vi "Do_Offset.vi"(0 "VRN IN":refnum<visa-resource-name>[](array[refnum])=["-1", "-1"] caption="VRN IN [TCS, Table, Prams]", 1 "TCS Actif":refnum<vi>, 2 "Table_Astrom":T2={"NAXIS"=[1000000.0, 1000000.0], "CD"=[[7.753782961940616e-07, 4.45891648260791e-07], [4.45891648260791e-07, -7.753782961940616e-07]], "CDELT"=[1.0, 1.0], "CRPIX"=[669354.0, 53563.0], "CTYPE"=["RA---TAN", "DEC--TAN"], "CRVAL"=[53.2938, 45.43681200000001], "LONGPOLE"=180.0, "LATPOLE"=90.0, "PV2"=[0.0, 0.0]} {"CRVAL" format="%.6g"; "CD" format="%_7g"}, 5 "RA offset":dbl format="%.2f", 9 "DEC offset":dbl format="%.2f", 11 "Error IN":errorcluster[](array[cluster])=[{"status"=FALSE, "code"=0, "source"=""}, {"status"=FALSE, "code"=0, "source"=""}] caption="Error IN [TCS C, Table]", 13 "Field_Astrom":T2 {"CRVAL" format="%.6g"; "CD" format="%_7g"}) -> (4 "VRN OUT":refnum<visa-resource-name>[](array[refnum]) caption="VRN OUT [TCS C, Table, Prams]", 6 "Error code":u8, 8 "Undo offset":bool, 10 "Warning code":u8, 14 "Error Comment":string, 15 "Error OUT":errorcluster[](array[cluster]) caption="Error OUT [TCS C, Table]")   [LabVIEW 2011]
uses:
  Globals.vi
  Polymorphics/Distance(array).vi
panel:
  out "BooleanReferences":T1
  out "Prams Error":errorcluster
  out "Table Error":errorcluster
  out "TCS Error":errorcluster
  in  "Prams VRN":refnum<visa-resource-name>
  in  "Table VRN":refnum<visa-resource-name>
  in  "TCS VRN":refnum<visa-resource-name>
  in  "Prams ACK":refnum<vi>
  in  "Prams Actif":refnum<vi>
  in  "Table Actif":refnum<vi>
  in  "FOV":dbl format="%.2f"
  in  "EPOCH":dbl format="%.2f"
  out "RA after":dbl
  out "DEC after":dbl
  in  "USNO_data":string[][](array[string])
  out "New Source Found ?":bool
  out "cible Y":dbl
  out "cible X":dbl
  out "Accesible?":bool
  out "DEC Goffset":dbl=10.0 format="%.2f"
  out "RA Goffset":dbl=10.0 format="%.2f"
  out "DEC Moffset":dbl format="%.2f"
  out "RA Moffset":dbl format="%.2f"
  out "Guiding":bool caption="Guider was running"
  out "Moffset":bool
  out "Goffset":bool
  out "Undo startguide":bool
  in  "goto accel":u32=200 max=1000
  in  "goto vite":u32=30000 min=1 max=500000
  in  "goto lent":u32=200 min=1 max=500000
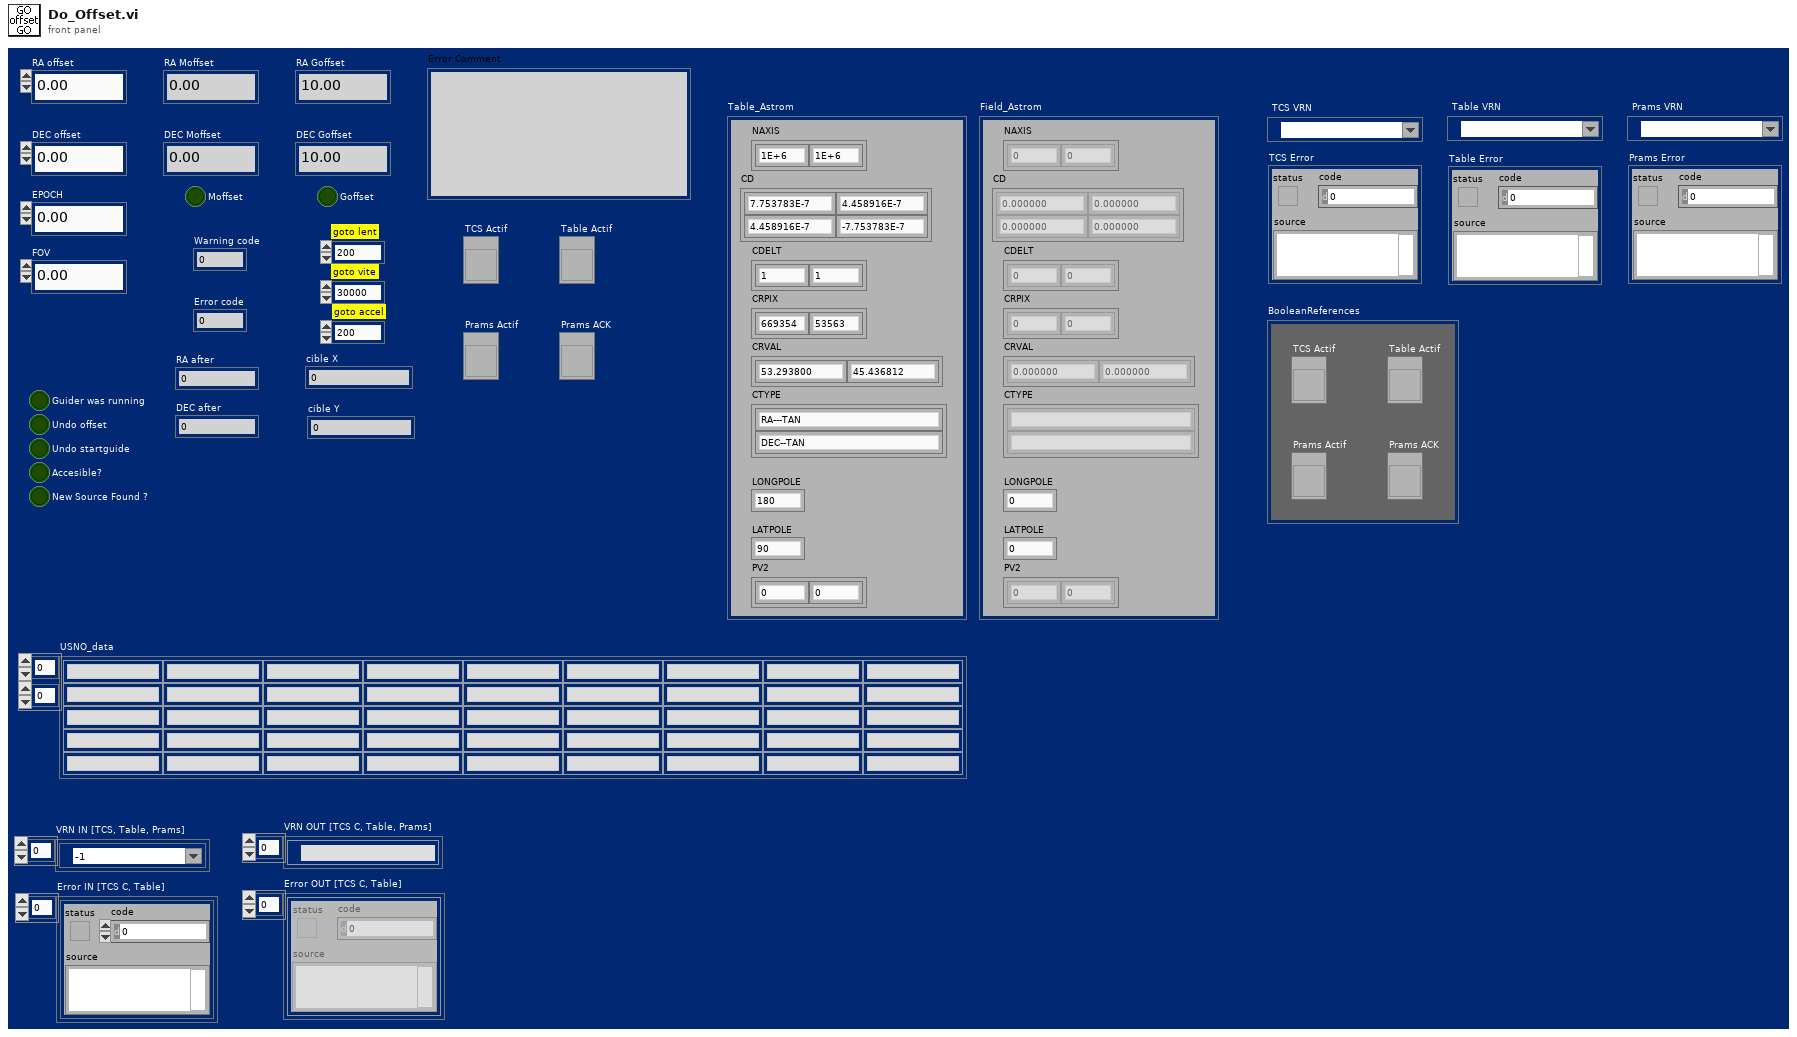
[diagram p1: front panel]
types:
  T1 = cluster{"TCS Actif":refnum<vi>, "Table Actif":refnum<vi>, "Prams Actif":refnum<vi>, "Prams ACK":refnum<vi>}
  T2 = cluster{"NAXIS":dbl[], "CD":dbl[][], "CDELT":dbl[], "CRPIX":dbl[], "CTYPE":string[], "CRVAL":dbl[], "LONGPOLE":dbl, "LATPOLE":dbl, "PV2":dbl[]}
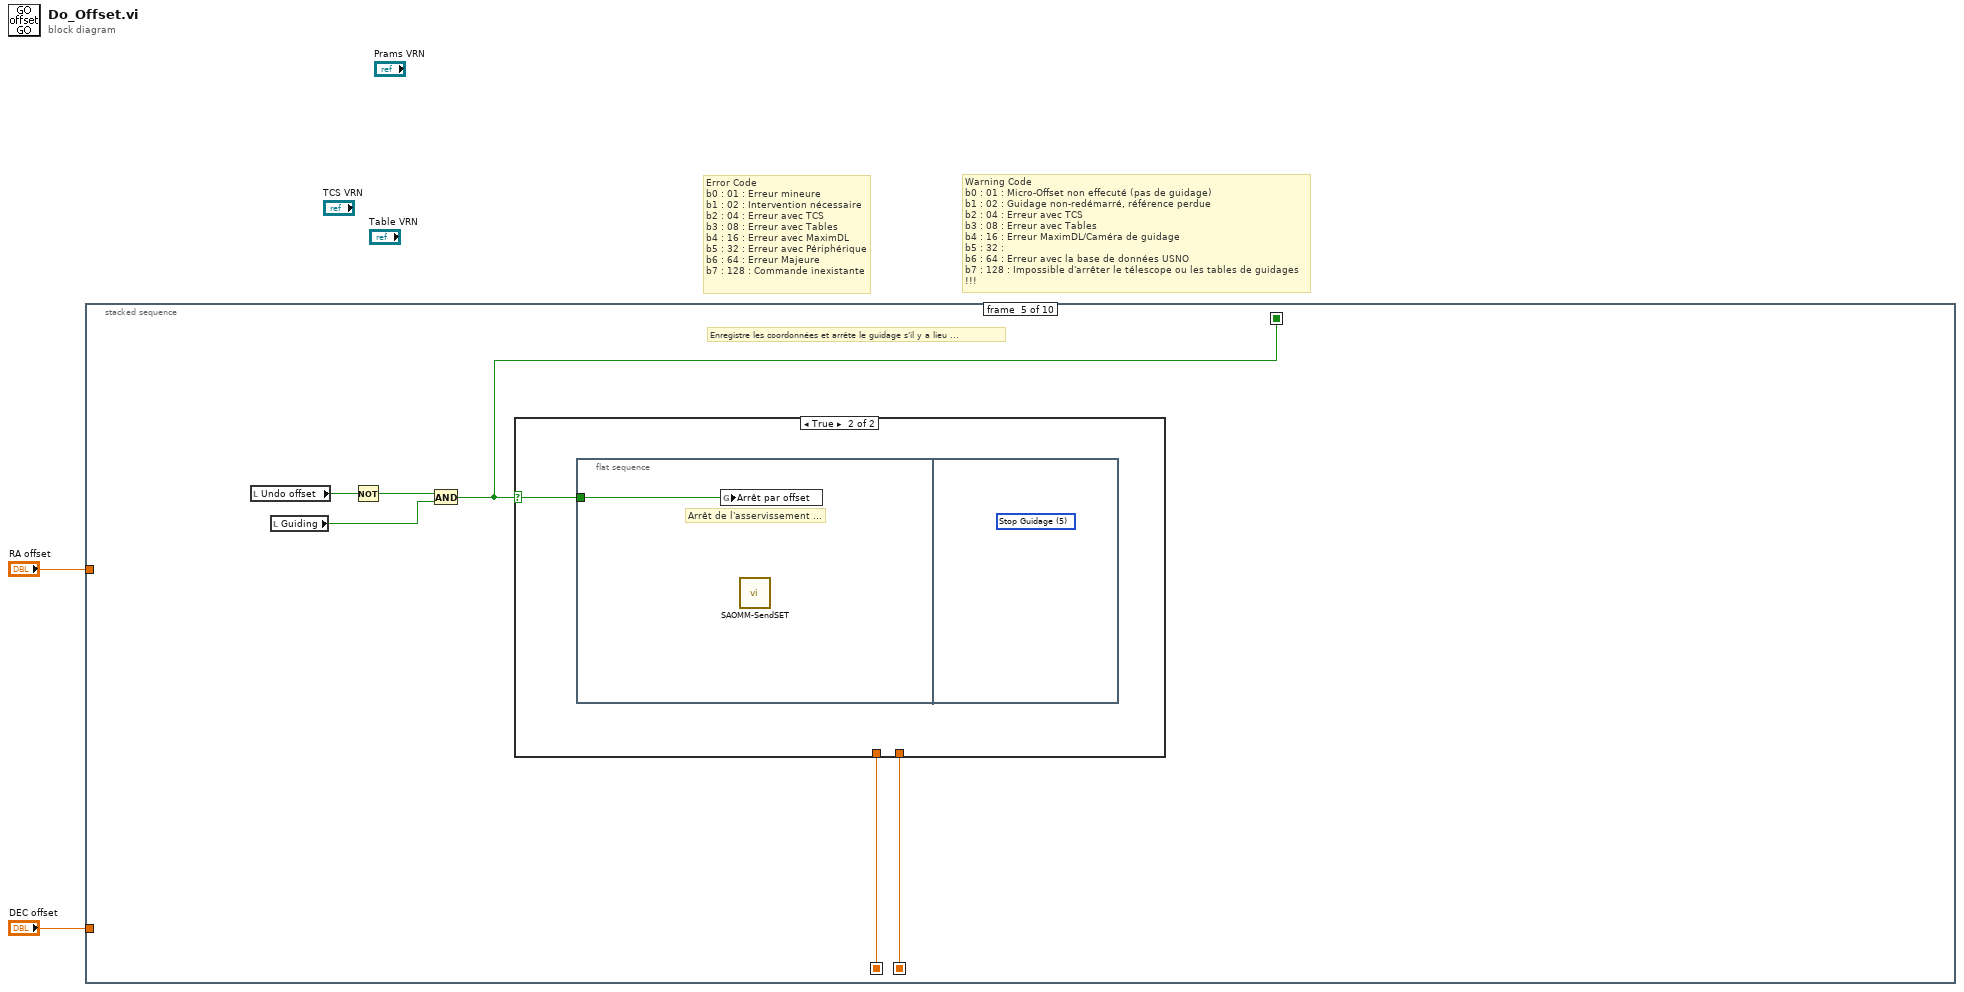
[diagram p0: block diagram]
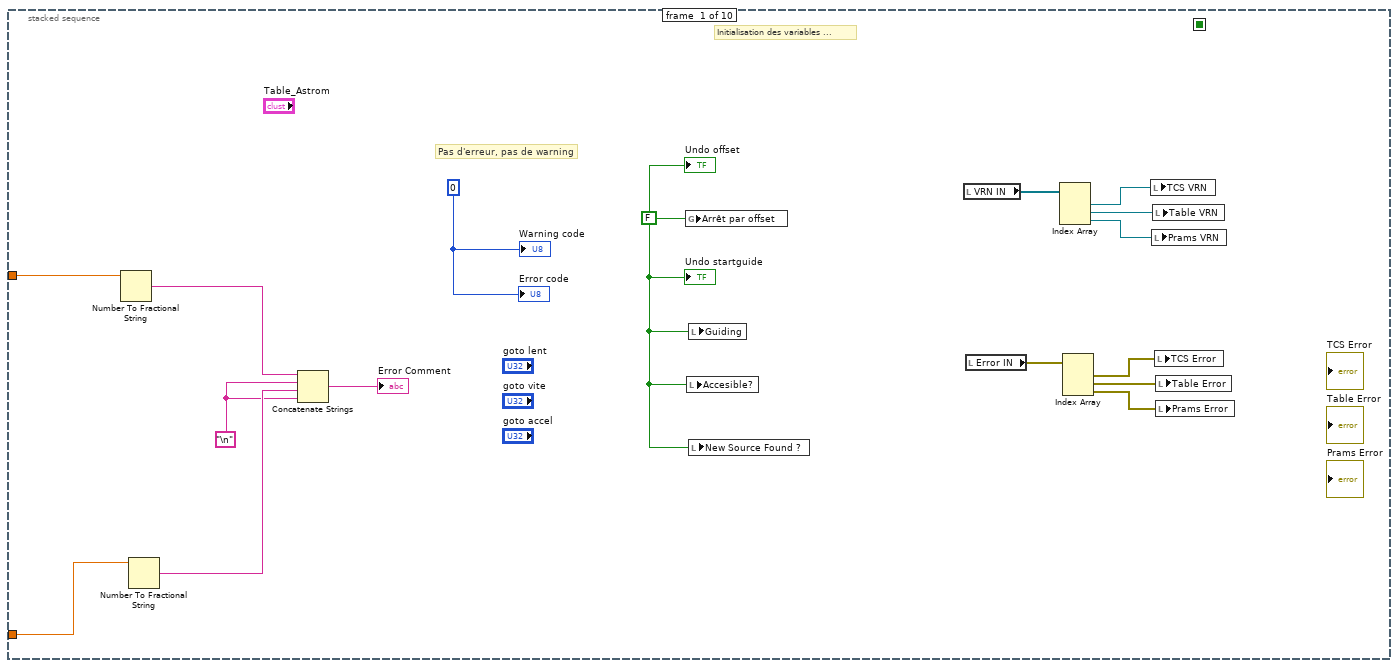
[diagram p2: hidden frame]
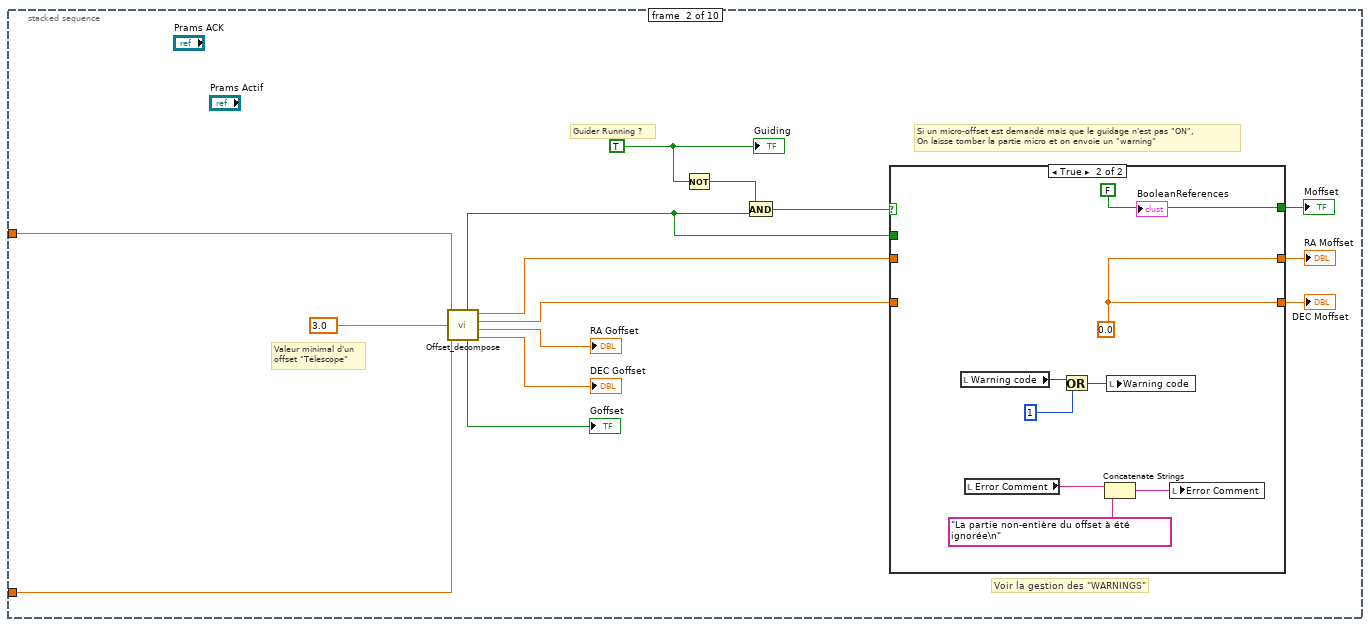
[diagram p3: hidden frame]
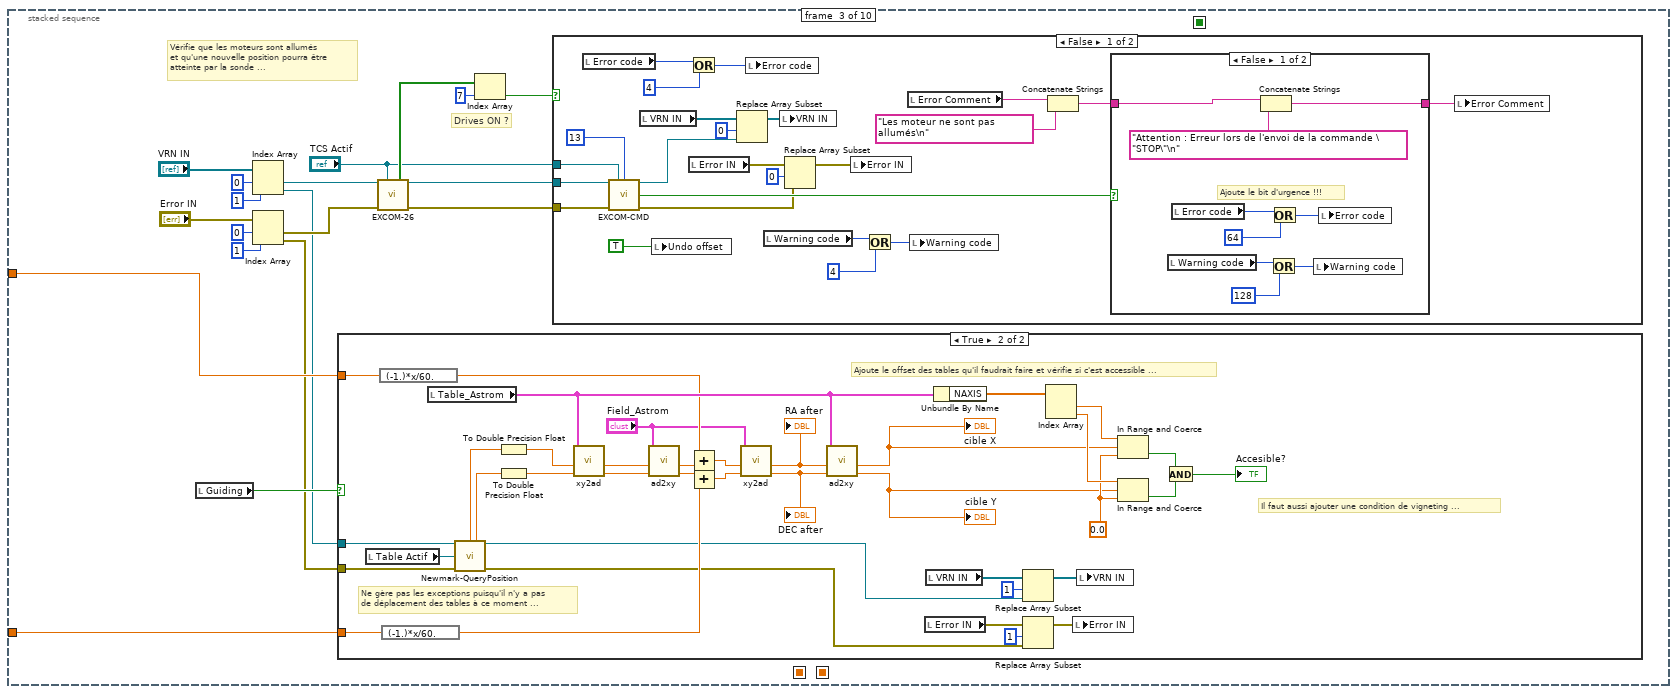
[diagram p5: hidden frame]
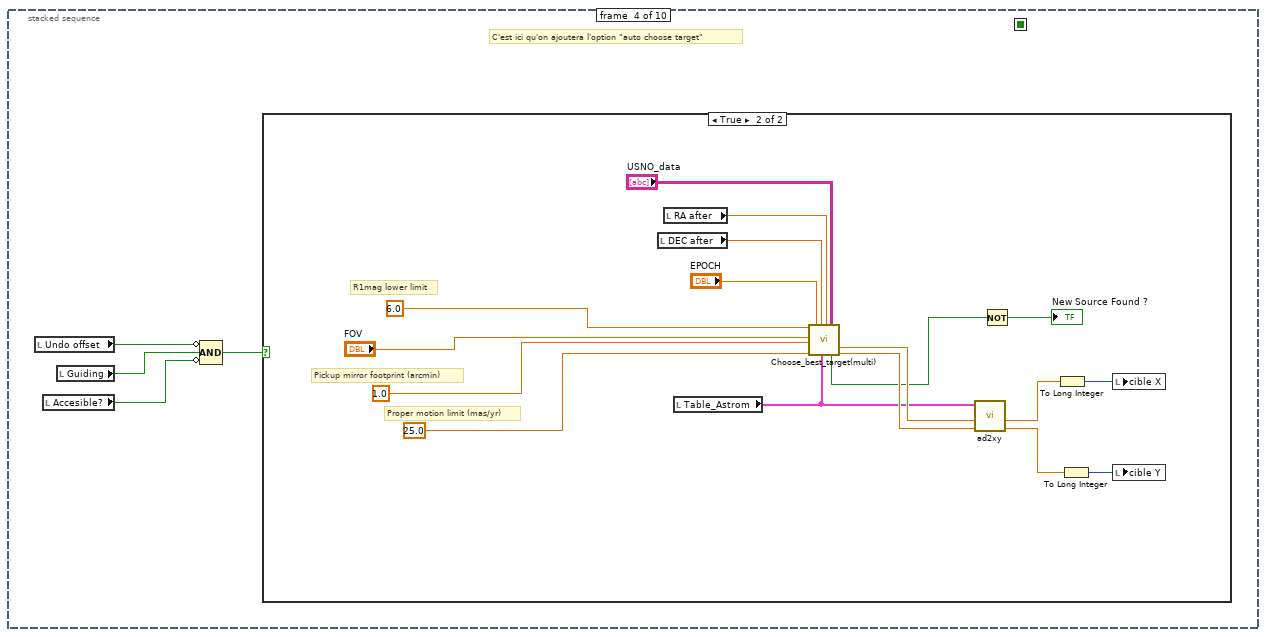
[diagram p9: hidden frame]
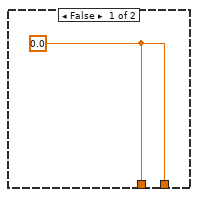
[diagram p11: hidden frame]
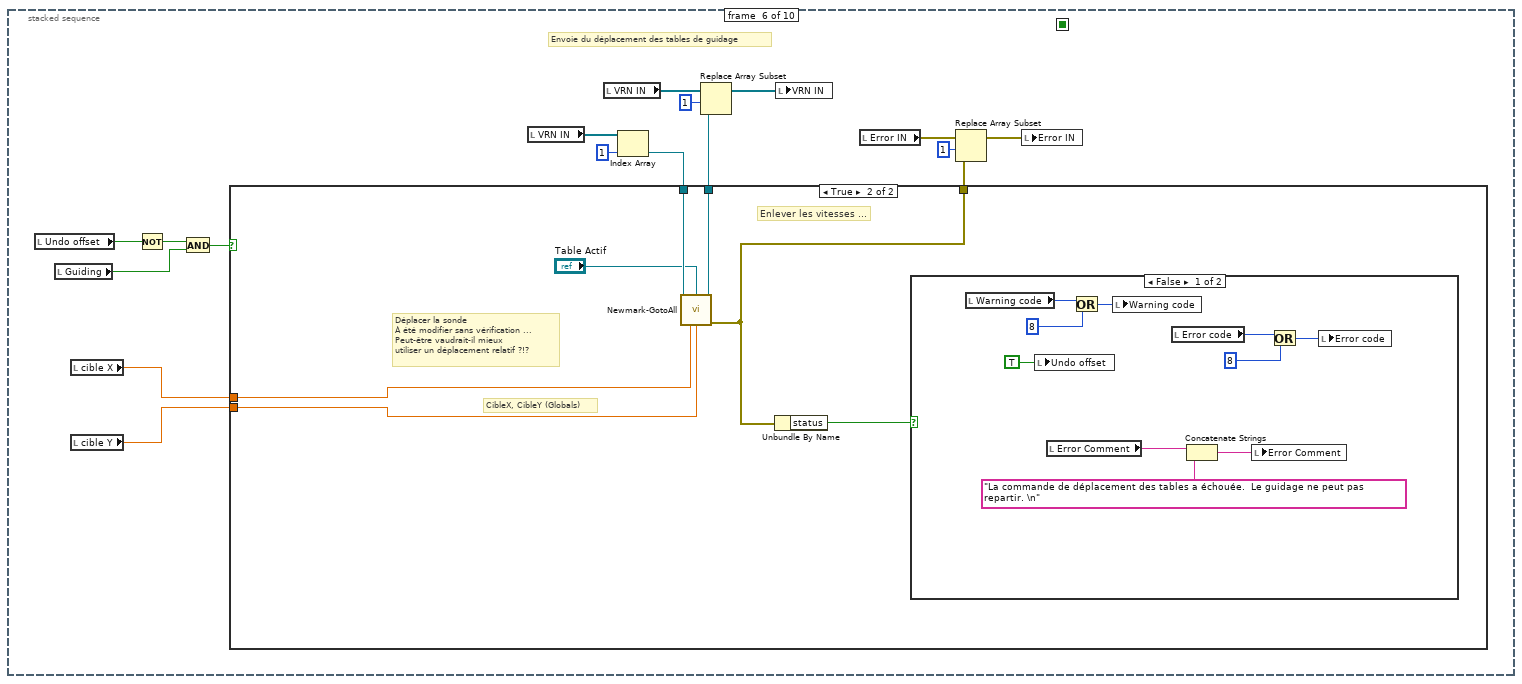
[diagram p12: hidden frame]
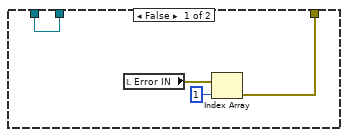
[diagram p13: hidden frame]
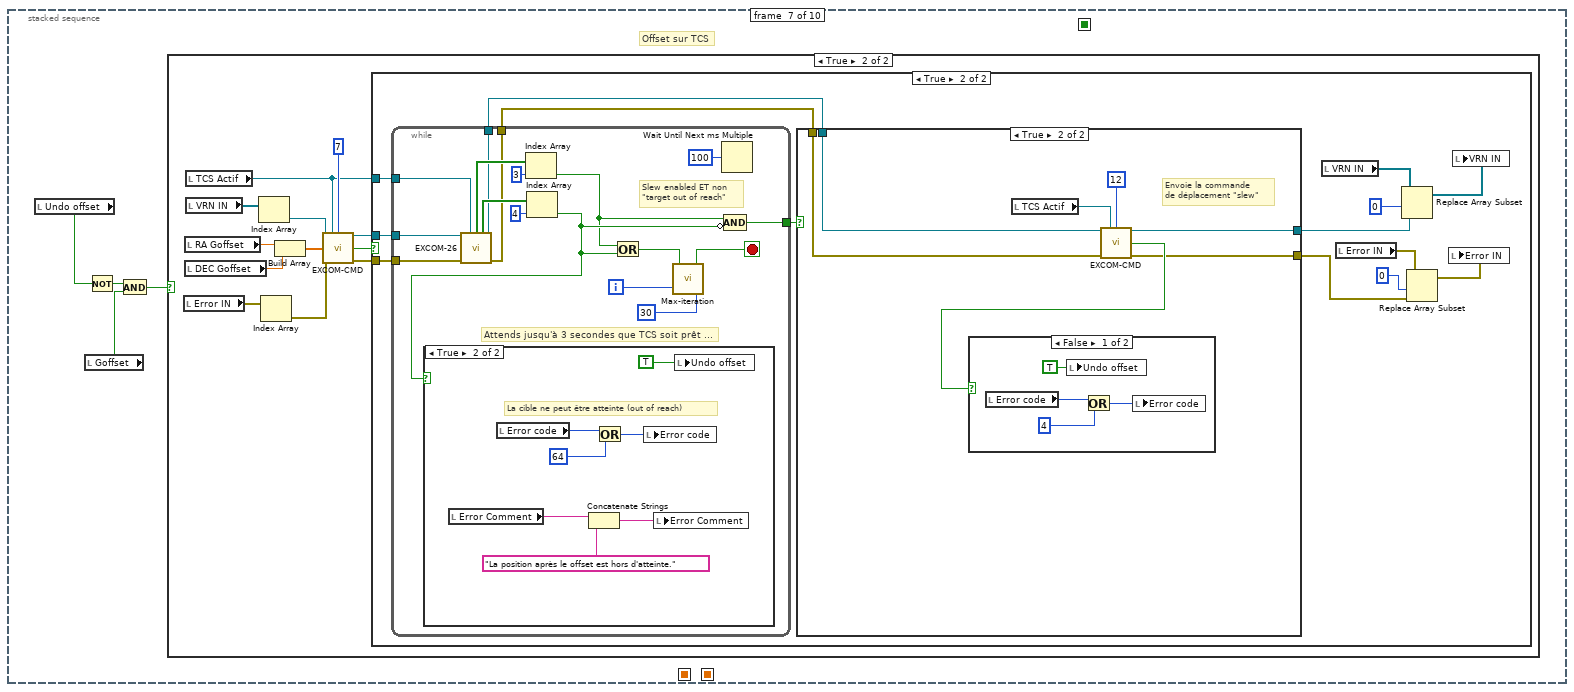
[diagram p15: hidden frame]
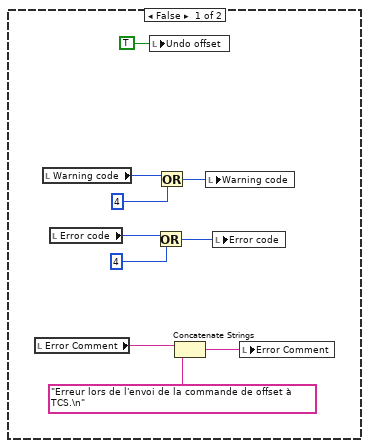
[diagram p17: hidden frame]
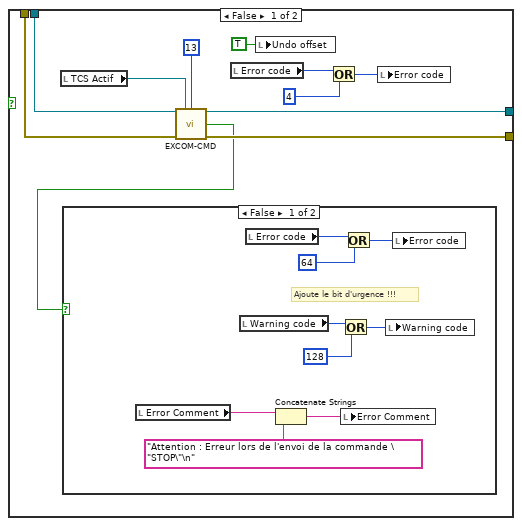
[diagram p19: hidden frame]
diagram:
  # "Error Code\nb0 : 01 : Erreur mineure\nb1 : 02 : Intervention nécessaire\nb2 : 04 : Erreur avec TCS\nb3 : 08 : Erreur avec Tables\nb4 : 16 : Erreur avec MaximDL\nb5 : 32 : Erreur avec Périphérique\nb6 : 64 : Erreur Majeure\nb7 : 128 : Commande inexistante"
  # "Warning Code\nb0 : 01 : Micro-Offset non effecuté (pas de guidage)\nb1 : 02 : Guidage non-redémarré, référence perdue\nb2 : 04 : Erreur avec TCS\nb3 : 08 : Erreur avec Tables\nb4 : 16 : Erreur MaximDL/Caméra de guidage\nb5 : 32 : \nb6 : 64 : Erreur avec la base de données USNO\nb7 : 128 : Impossible d'arrêter le télescope ou les tables de guidages !!!"
  n1 = stacked-sequence {
    seq-local: [_ _ _ _ w159 _ _ _ _ _] -> [_ _ _ _ _ _ _ _ _ _]
    seq-local: [_ _ _ _ w158 _ _ _ _ _] -> [_ _ _ _ _ _ _ _ w431 _]
    seq-local: [_ _ _ _ w157 _ _ _ _ _] -> [_ _ _ _ _ _ _ _ w430 _]
    tunnel: "DEC offset" -> [w15 w32 w61 _ _ _ _ _ _ _]
    tunnel: "RA offset" -> [w16 w33 w60 _ _ _ _ _ _ _]
    frame #0 {
      w11 = "\n"
      w17 = FALSE
      w18 = u8 0
      # "Initialisation des variables ..."
      # "Pas d'erreur, pas de warning"
      n2 = Number To Fractional String(number=w16) -> (F-format string=w14:string)  [unwired: 3 in]
      n3 = Number To Fractional String(number=w15) -> (F-format string=w13:string)  [unwired: 3 in]
      n4 = Concatenate Strings(w14, w11, w13, w11) -> (→"Error Comment":string)
      n5 = global write "Globals.vi" "Arrêt par offset"(w17) -> ()
      n6 = local write "Accesible?"(w17) -> ()
      n7 = local write "Guiding"(w17) -> ()
      n8 = local write "New Source Found ?"(w17) -> ()
      n9 = local read "VRN IN"() -> (w10:refnum<visa-resource-name>[])
      n10 = local read "Error IN"() -> (w9:errorcluster[])
      n11 = Index Array(array=w10) -> (element #1=w3:refnum<visa-resource-name>, element #2=w4:refnum<visa-resource-name>, element #3=w5:refnum<visa-resource-name>)  [unwired: 3 in]
      n12 = Index Array(array=w9) -> (element #1=w7:errorcluster, element #2=w8:errorcluster, element #3=w6:errorcluster)  [unwired: 3 in]
      n13 = local write "TCS VRN"(w3) -> ()
      n14 = local write "Prams VRN"(w5) -> ()
      n15 = local write "Table VRN"(w4) -> ()
      n16 = local write "TCS Error"(w7) -> ()
      n17 = local write "Table Error"(w8) -> ()
      n18 = local write "Prams Error"(w6) -> ()
      "Error code" <- w18
      "Warning code" <- w18
      "Undo offset" <- w17
      "Undo startguide" <- w17
    }
    frame #1 {
      w19 = TRUE
      # "Guider Running ?"
      # "Voir la gestion des \"WARNINGS\""
      # "Si un micro-offset est demandé mais que le guidage n'est pas \"ON\",\nOn laisse tomber la partie micro et on envoie un \"warning\""
      # "Valeur minimal d'un\noffset \"Télescope\""
      n19 = call "Offset_decompose.vi"("DEC offset"=w32, "RA offset"=w33, "Micro Limit"=3.0 ("y")) -> ("Goffset"=→"Goffset":bool, "Moffset"=w22:bool, "DEC Goffset"=→"DEC Goffset":dbl, "RA Goffset"=→"RA Goffset":dbl, "DEC Moffset"=w26:dbl, "RA Moffset"=w27:dbl)  [unwired: 2 in]
      n20 = Not(x=w19) -> (.not. x?=w28:bool)
      n21 = And(x=w28, y=w22) -> (x .and. y?=w23:bool)
      n22 = case shown="True" w23 {
        tunnel: w27 -> [w36 _]
        tunnel: w26 -> [w35 _]
        tunnel: [w36 w43] -> w25
        tunnel: [w35 w43] -> w24
        tunnel: w22 -> [w34 _]
        tunnel: [w34 FALSE] -> w20
        frame False {
        }
        frame True {
          w43 = 0.0
          n23 = local read "Warning code"() -> (w42:u8)
          n24 = local read "Error Comment"() -> (w39:string)
          n25 = Or(x=w42, y=u8 1) -> (x .or. y?=w41:u8)
          n26 = Concatenate Strings(w39, "La partie non-entière du offset à été ignorée\n") -> (w38:string)
          n27 = local write "Warning code"(w41) -> ()
          n28 = local write "Error Comment"(w38) -> ()
        }
      }
      "DEC Moffset" <- w24
      "RA Moffset" <- w25
      "Moffset" <- w20
      "Guiding" <- w19
    }
    frame #2 {
      # "Drives ON ?"
      # "Vérifie que les moteurs sont allumés\net qu'une nouvelle position pourra être\natteinte par la sonde ..."
      n29 = local read "Guiding"() -> (w59:bool)
      n30 = Index Array(array="VRN IN", index #1=0 ("index"), index #2=1 ("index")) -> (element #1=w50:refnum<visa-resource-name>, element #2=w47:refnum<visa-resource-name>)
      n31 = Index Array(array="Error IN", index #1=0 ("index"), index #2=1 ("index")) -> (element #1=w54:errorcluster, element #2=w45:errorcluster)
      n32 = case shown="True" w59 {
        tunnel: w61 -> [_ w99]
        tunnel: w60 -> [_ w98]
        tunnel: w47 -> [_ w73]
        tunnel: w45 -> [_ w72]
        frame False {
        }
        frame True {
          w91 = 0.0
          # "Ne gère pas les exceptions puisqu'il n'y a pas\nde déplacement des tables à ce moment ..."
          # "Il faut aussi ajouter une condition de vigneting ..."
          # "Ajoute le offset des tables qu'il faudrait faire et vérifie si c'est accessible ..."
          n33 = local read "Table Actif"() -> (w74:refnum<vi>)
          n34 = expression code="(-1.)*x/60."(w98) -> (w85:dbl)
          n35 = expression code="(-1.)*x/60."(w99) -> (w84:dbl)
          n36 = local read "Table_Astrom"() -> (w97:T2)
          n37 = call "Newmark-QueryPosition.vi"("Table VRN IN"=w73, "Bool Refnum"=w74, "Error IN"=w72) -> ("X Axis"=w76:dbl, "Y Axis"=w75:dbl, "Table VRN OUT"=w65:refnum<visa-resource-name>, "Error OUT"=w64:errorcluster)  [unwired: 5 in, 4 out]
          n38 = To Double Precision Float(number=w76) -> (double precision float=w101:dbl)
          n39 = To Double Precision Float(number=w75) -> (double precision float=w100:dbl)
          n40 = call "xy2ad.vi"("Y (px)"=w100, "X (px)"=w101, "Astrometry"=w97) -> ("DEC (°)"=w88:dbl, "RA (°)"=w89:dbl)  [unwired: 5 in, 2 out]
          n41 = call "ad2xy.vi"("DEC"=w88, "RA"=w89, "Astrometry"="Field_Astrom") -> ("Y"=w86:dbl, "X"=w87:dbl)  [unwired: 6 in, 1 out]
          n42 = Add(x=w85, y=w87) -> (x+y=w83:dbl)
          n43 = Add(x=w86, y=w84) -> (x+y=w82:dbl)
          n44 = call "xy2ad.vi"("Y (px)"=w82, "X (px)"=w83, "Astrometry"="Field_Astrom") -> ("DEC (°)"=w80:dbl, "RA (°)"=w81:dbl)  [unwired: 5 in, 2 out]
          "DEC after" <- w80
          "RA after" <- w81
          n45 = call "ad2xy.vi"("DEC"=w80, "RA"=w81, "Astrometry"=w97) -> ("Y"=w77:dbl, "X"=w78:dbl)  [unwired: 6 in, 1 out]
          "cible X" <- w78
          "cible Y" <- w77
          n46 = local read "Error IN"() -> (w70:errorcluster[])
          n47 = local read "VRN IN"() -> (w67:refnum<visa-resource-name>[])
          n48 = Unbundle By Name(w97) -> ("NAXIS"=w96:dbl[])
          n49 = Replace Array Subset(array=w67, new element=w65, index=1) -> (w66:refnum<visa-resource-name>[])
          n50 = Replace Array Subset(array=w70, new element=w64, index=1) -> (w71:errorcluster[])
          n51 = Index Array(array=w96) -> (element #1=w95:dbl, element #2=w94:dbl)  [unwired: 2 in]
          n52 = local write "Error IN"(w71) -> ()
          n53 = local write "VRN IN"(w66) -> ()
          n54 = In Range and Coerce(upper limit=w95, x=w78, lower limit=w91) -> (In Range?=w93:bool)  [unwired: 1 out]
          n55 = In Range and Coerce(upper limit=w94, x=w77, lower limit=w91) -> (In Range?=w92:bool)  [unwired: 1 out]
          n56 = And(x=w93, y=w92) -> (x .and. y?=→"Accesible?":bool)
        }
      }
      n57 = call "EXCOM-26.vi"("VRN IN"=w50, "Bool Refnum"="TCS Actif", "Error IN"=w54) -> ("STATH"=w57:bool[], "VRN OUT"=w62:refnum<visa-resource-name>, "Error OUT"=w56:errorcluster)  [unwired: 6 in, 4 out]
      n58 = Index Array(array=w57, index=7 ("Index")) -> (element=w63:bool)
      n59 = case shown="False" w63 {
        tunnel: w62 -> [w120 _]
        tunnel: w56 -> [w115 _]
        tunnel: "TCS Actif" -> [w106 _]
        frame False {
          n60 = local read "Error code"() -> (w125:u8)
          n61 = call "EXCOM-CMD.vi"("VRN IN"=w120, "Bool Refnum"=w106, "Commande #"=13 ("NombredArguments"), "Error IN"=w115) -> ("VRN OUT"=w113:refnum<visa-resource-name>, "OK Done"=w121:bool, "Error OUT"=w110:errorcluster)  [unwired: 9 in]
          n62 = local read "VRN IN"() -> (w112:refnum<visa-resource-name>[])
          n63 = local write "Undo offset"(TRUE) -> ()
          n64 = Or(x=w125, y=u8 4) -> (x .or. y?=w124:u8)
          n65 = local read "Error IN"() -> (w108:errorcluster[])
          n66 = Replace Array Subset(array=w112, new element=w113, index=0) -> (w114:refnum<visa-resource-name>[])
          n67 = local write "Error code"(w124) -> ()
          n68 = local read "Warning code"() -> (w119:u8)
          n69 = local write "VRN IN"(w114) -> ()
          n70 = Replace Array Subset(array=w108, new element=w110, index=0) -> (w107:errorcluster[])
          n71 = local write "Error IN"(w107) -> ()
          n72 = Or(x=w119, y=u8 4) -> (x .or. y?=w118:u8)
          n73 = local read "Error Comment"() -> (w105:string)
          n74 = local write "Warning code"(w118) -> ()
          n75 = Concatenate Strings(w105, "Les moteur ne sont pas allumés\n") -> (w103:string)
          n76 = case shown="False" w121 {
            tunnel: w103 -> [w128 w135]
            tunnel: [w127 w135] -> w102
            frame False {
              # "Ajoute le bit d'urgence !!!"
              n77 = local read "Warning code"() -> (w132:u8)
              n78 = local read "Error code"() -> (w131:u8)
              n79 = Concatenate Strings(w128, "Attention : Erreur lors de l'envoi de la commande \"STOP\"\n" ("string")) -> (w127:string)
              n80 = Or(x=w132, y=u8 128) -> (x .or. y?=w133:u8)
              n81 = Or(x=w131, y=u8 64) -> (x .or. y?=w130:u8)
              n82 = local write "Warning code"(w133) -> ()
              n83 = local write "Error code"(w130) -> ()
            }
            frame True {
            }
          }
          n84 = local write "Error Comment"(w102) -> ()
        }
        frame True {
        }
      }
    }
    frame #3 {
      # "C'est ici qu'on ajoutera l'option \"auto choose target\""
      n85 = local read "Undo offset"() -> (w139:bool)
      n86 = local read "Accesible?"() -> (w137:bool)
      n87 = local read "Guiding"() -> (w138:bool)
      n88 = Compound Arithmetic op=AND(invert w139, w138, invert w137) -> (w136:bool)
      n89 = case shown="True" w136 {
        frame False {
        }
        frame True {
          # "Proper motion limit (mas/yr)"
          # "Pickup mirror footprint (arcmin)"
          # "R1mag lower limit"
          n90 = local read "DEC after"() -> (w155:dbl)
          n91 = local read "RA after"() -> (w156:dbl)
          n92 = local read "Table_Astrom"() -> (w146:T2)
          n93 = call "Choose_best_target(multi).vi"("R1mag lower limit"=6.0, "FOV"="FOV", "Footprint"=1.0, "PM limit"=25.0 ("Footprint"), "EPOCH TEL"="EPOCH", "DEC TEL"=w155, "Table Astrometry"=w146, "RA TEL"=w156, "USNO_data"="USNO_data") -> ("erreur"=w141:bool, "target RA (deg)"=w149:dbl, "target DEC (deg)"=w148:dbl)  [unwired: 3 in, 5 out]
          n94 = call "ad2xy.vi"("DEC"=w148, "RA"=w149, "Astrometry"=w146) -> ("Y"=w150:dbl, "X"=w151:dbl)  [unwired: 6 in, 1 out]
          n95 = Not(x=w141) -> (.not. x?=→"New Source Found ?":bool)
          n96 = To Long Integer(number=w151) -> (32bit integer=w153:i32)
          n97 = To Long Integer(number=w150) -> (32bit integer=w152:i32)
          n98 = local write "cible X"(w153) -> ()
          n99 = local write "cible Y"(w152) -> ()
        }
      }
    }
    frame #4 {
      # "Enregistre les coordonnées et arrête le guidage s'il y a lieu ..."
      n100 = local read "Undo offset"() -> (w161:bool)
      n101 = local read "Guiding"() -> (w160:bool)
      n102 = Not(x=w161) -> (.not. x?=w162:bool)
      n103 = And(x=w162, y=w160) -> (x .and. y?=w159:bool)
      n104 = case shown="True" w159 {
        selector: w159 -> [_ w164]
        tunnel: [w163 _] -> w157
        tunnel: [w163 _] -> w158
        frame False {
          w163 = sgl 0.0 ("GuiderYError")
        }
        frame True {
          n105 = flat-sequence {
            tunnel: w164 -> [w165]
            frame #0 {
              # "Arrêt de l'asservissement ..."
              n106 = global write "Globals.vi" "Arrêt par offset"(w165) -> ()
              n107 = call "SAOMM-SendSET.vi"() -> ()  [unwired: 12 in, 4 out]
            }
            frame #1 {
              (unwired) u16 5 items=["Exposition Guideur", "Calibration", "Guidage", "Piedestal", "Exposition simple", "Stop Guidage"] ("Mode")
            }
          }
        }
      }
    }
    frame #5 {
      # "Envoie du déplacement des tables de guidage"
      n108 = local read "Undo offset"() -> (w178:bool)
      n109 = local read "Guiding"() -> (w177:bool)
      n110 = local read "cible X"() -> (w182:dbl)
      n111 = local read "cible Y"() -> (w181:dbl)
      n112 = Not(x=w178) -> (.not. x?=w179:bool)
      n113 = And(x=w179, y=w177) -> (x .and. y?=w180:bool)
      n114 = local read "VRN IN"() -> (w174:refnum<visa-resource-name>[])
      n115 = local read "VRN IN"() -> (w172:refnum<visa-resource-name>[])
      n116 = Index Array(array=w174, index=1) -> (element=w175:refnum<visa-resource-name>)
      n117 = case shown="True" w180 {
        tunnel: w181 -> [_ w187]
        tunnel: w182 -> [_ w188]
        tunnel: w175 -> [w186 w193]
        tunnel: [w186 w192] -> w170
        tunnel: [w184 w191] -> w166
        frame False {
          n118 = local read "Error IN"() -> (w185:errorcluster[])
          n119 = Index Array(array=w185, index=1) -> (element=w184:errorcluster)
        }
        frame True {
          # "CibleX, CibleY (Globals)"
          # "Enlever les vitesses ..."
          # "Déplacer la sonde\nÀ été modifier sans vérification ...\nPeut-être vaudrait-il mieux\nutiliser un déplacement relatif ?!?"
          n120 = call "Newmark-GotoAll.vi"("Table VRN IN"=w193, "Bool Refnum"="Table Actif", "Position X"=w188, "Position Y"=w187) -> ("Table VRN OUT"=w192:refnum<visa-resource-name>, "Error OUT"=w191:errorcluster)  [unwired: 10 in]
          n121 = Unbundle By Name(w191) -> ("status"=w190:bool)
          n122 = case shown="False" w190 {
            frame False {
              n123 = local read "Warning code"() -> (w199:u8)
              n124 = local write "Undo offset"(TRUE) -> ()
              n125 = local read "Error Comment"() -> (w196:string)
              n126 = Or(x=w199, y=u8 8) -> (x .or. y?=w198:u8)
              n127 = local write "Warning code"(w198) -> ()
              n128 = local read "Error code"() -> (w200:u8)
              n129 = Concatenate Strings(w196, "La commande de déplacement des tables a échouée.  Le guidage ne peut pas repartir. \n") -> (w195:string)
              n130 = local write "Error Comment"(w195) -> ()
              n131 = Or(x=w200, y=u8 8) -> (x .or. y?=w201:u8)
              n132 = local write "Error code"(w201) -> ()
            }
            frame True {
            }
          }
        }
      }
      n133 = Replace Array Subset(array=w172, new element=w170, index=1) -> (w173:refnum<visa-resource-name>[])
      n134 = local write "VRN IN"(w173) -> ()
      n135 = local read "Error IN"() -> (w168:errorcluster[])
      n136 = Replace Array Subset(array=w168, new element=w166, index=1) -> (w167:errorcluster[])
      n137 = local write "Error IN"(w167) -> ()
    }
    frame #6 {
      # "Offset sur TCS"
      n138 = local read "Undo offset"() -> (w205:bool)
      n139 = local read "Goffset"() -> (w204:bool)
      n140 = Not(x=w205) -> (.not. x?=w206:bool)
      n141 = And(x=w206, y=w204) -> (x .and. y?=w207:bool)
      n142 = case shown="True" w207 {
        frame False {
        }
        frame True {
          n143 = local read "Error IN"() -> (w210:errorcluster[])
          n144 = local read "RA Goffset"() -> (w214:dbl)
          n145 = local read "DEC Goffset"() -> (w215:dbl)
          n146 = local read "TCS Actif"() -> (w208:refnum<vi>)
          n147 = local read "VRN IN"() -> (w212:refnum<visa-resource-name>[])
          n148 = Index Array(array=w212) -> (element=w211:refnum<visa-resource-name>)  [unwired: 1 in]
          n149 = Index Array(array=w210) -> (element=w209:errorcluster)  [unwired: 1 in]
          n150 = Build Array(w214, w215) -> (w213:dbl[])
          n151 = call "EXCOM-CMD.vi"("VRN IN"=w211, "Bool Refnum"=w208, "Commande #"=7 ("NombredArguments"), "Args"=w213, "Error IN"=w209) -> ("VRN OUT"=w218:refnum<visa-resource-name>, "OK Done"=w219:bool, "Error OUT"=w216:errorcluster)  [unwired: 8 in]
          n152 = case shown="True" w219 {
            tunnel: w218 -> [_ w242]
            tunnel: w216 -> [_ w240]
            tunnel: w208 -> [_ w230]
            frame False {
              n153 = local read "Error Comment"() -> (w222:string)
              n154 = local read "Warning code"() -> (w223:u8)
              n155 = local read "Error code"() -> (w228:u8)
              n156 = local write "Undo offset"(TRUE) -> ()
              n157 = Or(x=w228, y=u8 4) -> (x .or. y?=w227:u8)
              n158 = Or(x=w223, y=u8 4) -> (x .or. y?=w224:u8)
              n159 = Concatenate Strings(w222, "Erreur lors de l'envoi de la commande de offset à TCS.\n") -> (w221:string)
              n160 = local write "Warning code"(w224) -> ()
              n161 = local write "Error code"(w227) -> ()
              n162 = local write "Error Comment"(w221) -> ()
            }
            frame True {
              n163 = while {
                tunnel: [w247] -> w243
                tunnel: w242 -> [w255]
                tunnel: [w254] -> w241
                tunnel: w240 -> [w246]
                tunnel: [w245] -> w239
                tunnel: w230 -> [w244]
                i -> [w251]
                stop <- w252 stop-if-true
                # "Slew enabled ET non\n\"target out of reach\""
                # "Attends jusqu'à 3 secondes que TCS soit prêt ..."
                n164 = call "EXCOM-26.vi"("VRN IN"=w255, "Bool Refnum"=w244, "Error IN"=w246) -> ("STATL"=w257:bool[], "STATH"=w256:bool[], "VRN OUT"=w254:refnum<visa-resource-name>, "Error OUT"=w245:errorcluster)  [unwired: 6 in, 3 out]
                n165 = Index Array(array=w257, index=3 ("Index")) -> (element=w248:bool)
                n166 = Index Array(array=w256, index=4 ("Index")) -> (element=w249:bool)
                n167 = case shown="True" w249 {
                  frame False {
                  }
                  frame True {
                    # "La cible ne peut être atteinte (out of reach)"
                    n168 = local read "Error Comment"() -> (w263:string)
                    n169 = local read "Error code"() -> (w267:u8)
                    n170 = Concatenate Strings(w263, "La position après le offset est hors d'atteinte.") -> (w262:string)
                    n171 = Or(x=w267, y=u8 64) -> (x .or. y?=w266:u8)
                    n172 = local write "Error code"(w266) -> ()
                    n173 = local write "Error Comment"(w262) -> ()
                    n174 = local write "Undo offset"(TRUE ("Undo offset")) -> ()
                  }
                }
                n175 = Or(x=w248, y=w249) -> (x .or. y?=w253:bool)
                n176 = call "Max-iteration.vi"("i max"=30, "i act"=w251, "Valeur entrante"=w253) -> ("break ?"=w252:bool)
                n177 = Wait Until Next ms Multiple(millisecond multiple=u32 100 ("n millisecondes")) -> ()  [unwired: 1 out]
                n178 = Compound Arithmetic op=AND(w248, invert w249) -> (w247:bool)
              }
              n179 = case shown="True" w243 {
                tunnel: w241 -> [w277 w294]
                tunnel: [w272 w291] -> w235
                tunnel: w239 -> [w271 w290]
                tunnel: [w270 w289] -> w236
                frame False {
                  n180 = local read "TCS Actif"() -> (w269:refnum<vi>)
                  n181 = call "EXCOM-CMD.vi"("VRN IN"=w277, "Bool Refnum"=w269, "Commande #"=13 ("NombredArguments"), "Error IN"=w271) -> ("VRN OUT"=w272:refnum<visa-resource-name>, "OK Done"=w268:bool, "Error OUT"=w270:errorcluster)  [unwired: 9 in]
                  n182 = case shown="False" w268 {
                    frame False {
                      # "Ajoute le bit d'urgence !!!"
                      n183 = local read "Error Comment"() -> (w281:string)
                      n184 = local read "Warning code"() -> (w285:u8)
                      n185 = local read "Error code"() -> (w284:u8)
                      n186 = Concatenate Strings(w281, "Attention : Erreur lors de l'envoi de la commande \"STOP\"\n" ("string")) -> (w280:string)
                      n187 = Or(x=w285, y=u8 128) -> (x .or. y?=w286:u8)
                      n188 = local write "Error Comment"(w280) -> ()
                      n189 = Or(x=w284, y=u8 64) -> (x .or. y?=w283:u8)
                      n190 = local write "Warning code"(w286) -> ()
                      n191 = local write "Error code"(w283) -> ()
                    }
                    frame True {
                    }
                  }
                  n192 = local read "Error code"() -> (w274:u8)
                  n193 = local write "Undo offset"(TRUE ("Undo offset")) -> ()
                  n194 = Or(x=w274, y=u8 4) -> (x .or. y?=w275:u8)
                  n195 = local write "Error code"(w275) -> ()
                }
                frame True {
                  # "Envoie la commande\nde déplacement \"slew\""
                  n196 = local read "TCS Actif"() -> (w288:refnum<vi>)
                  n197 = call "EXCOM-CMD.vi"("VRN IN"=w294, "Bool Refnum"=w288, "Commande #"=12, "Error IN"=w290) -> ("VRN OUT"=w291:refnum<visa-resource-name>, "OK Done"=w293:bool, "Error OUT"=w289:errorcluster)  [unwired: 9 in]
                  n198 = case shown="False" w293 {
                    frame False {
                      n199 = local read "Error code"() -> (w296:u8)
                      n200 = local write "Undo offset"(TRUE ("Undo offset")) -> ()
                      n201 = Or(x=w296, y=u8 4) -> (x .or. y?=w297:u8)
                      n202 = local write "Error code"(w297) -> ()
                    }
                    frame True {
                    }
                  }
                }
              }
              n203 = local read "VRN IN"() -> (w234:refnum<visa-resource-name>[])
              n204 = local read "Error IN"() -> (w233:errorcluster[])
              n205 = Replace Array Subset(array=w234, new element=w235, index=0) -> (w237:refnum<visa-resource-name>[])
              n206 = Replace Array Subset(array=w233, new element=w236, index=0) -> (w238:errorcluster[])
              n207 = local write "Error IN"(w238) -> ()
              n208 = local write "VRN IN"(w237) -> ()
            }
          }
        }
      }
    }
    frame #7 {
      # "Attends que tous les déplacement soit complétés ..."
      n209 = local read "Undo offset"() -> (w299:bool)
      n210 = case shown="False" w299 {
        frame False {
          # "If NOT Monitor Table AND $\nGuiding AND NOT $\n\"Undo StartGuide\" $\nTHEN StartGuide"
          # "Ajoute les codes d'erreurs correspondants et arrête le Télescope"
          # "Attends jusqu'à 30 secondes que \"SLEW\" redevienne \"OFF\""
          # "Attends 3 sec que \"SLEW\" soit \"ON\"\nVérifier qu'il n'y a pas des cas où le\nmouvement se fait sans que le flag monte ..."
          # "Si vrai, il y a eu une erreur ..."
          n211 = local read "Error IN"() -> (w318:errorcluster[])
          n212 = local read "VRN IN"() -> (w317:refnum<visa-resource-name>[])
          n213 = local read "TCS Actif"() -> (w305:refnum<vi>)
          n214 = Index Array(array=w317) -> (element=w316:refnum<visa-resource-name>)  [unwired: 1 in]
          n215 = Index Array(array=w318) -> (element=w315:errorcluster)  [unwired: 1 in]
          n216 = while {
            tunnel: [w423] -> w302
            i -> [w427]
            stop <- w426 stop-if-true
            w423 = FALSE
            # "Devra être changer quand on décidera de la\nfaçon de gérer le déplacement des tables ..."
            # "Attends jusqu'à 30 secondes après les tables"
            n217 = Not(x=w423) -> (.not. x?=w424:bool)
            n218 = call "Max-iteration.vi"("i max"=300, "i act"=w427, "Valeur entrante"=w424) -> ("break ?"=w426:bool)
            n219 = Wait Until Next ms Multiple(millisecond multiple=u32 200) -> ()  [unwired: 1 out]
          }
          n220 = while {
            tunnel: [w422] -> w325
            tunnel: w316 -> [w421]
            tunnel: [w414] -> w324
            tunnel: [w413] -> w320
            tunnel: w315 -> [w412]
            tunnel: w305 -> [w411]
            tunnel: [w411] -> w304
            i -> [w417]
            stop <- w415 stop-if-true
            n221 = call "EXCOM-26.vi"("VRN IN"=w421, "Bool Refnum"=w411, "Error IN"=w412) -> ("STATL"=w419:bool[], "VRN OUT"=w422:refnum<visa-resource-name>, "Error OUT"=w413:errorcluster)  [unwired: 6 in, 4 out]
            n222 = Wait Until Next ms Multiple(millisecond multiple=u32 100 ("n millisecondes")) -> ()  [unwired: 1 out]
            n223 = Index Array(array=w419, index=7 ("Index")) -> (element=w414:bool)
            n224 = call "Max-iteration.vi"("i max"=30, "i act"=w417, "Valeur entrante"=w414) -> ("break ?"=w415:bool)
          }
          n225 = case shown="True" w324 {
            selector: w324 -> [w390 _]
            tunnel: w325 -> [w389 w397]
            tunnel: [w390 w396] -> w323
            tunnel: w320 -> [w388 w395]
            tunnel: [w389 w394] -> w319
            tunnel: [w388 w393] -> w314
            tunnel: w304 -> [w387 w392]
            tunnel: [w387 w391] -> w303
            frame False {
            }
            frame True {
              n226 = while {
                tunnel: w397 -> [w407]
                tunnel: [w402] -> w396
                tunnel: w395 -> [w401]
                tunnel: [w400] -> w393
                tunnel: [w399] -> w394
                tunnel: w392 -> [w398]
                tunnel: [w398] -> w391
                i -> [w404]
                stop <- w403 stop-if-true
                n227 = call "EXCOM-26.vi"("VRN IN"=w407, "Bool Refnum"=w398, "Error IN"=w401) -> ("STATL"=w408:bool[], "VRN OUT"=w399:refnum<visa-resource-name>, "Error OUT"=w400:errorcluster)  [unwired: 6 in, 4 out]
                n228 = Index Array(array=w408, index=7 ("Index")) -> (element=w409:bool)
                n229 = Wait Until Next ms Multiple(millisecond multiple=u32 100 ("n millisecondes")) -> ()  [unwired: 1 out]
                n230 = Not(x=w409) -> (.not. x?=w402:bool)
                n231 = call "Max-iteration.vi"("i max"=300, "i act"=w404, "Valeur entrante"=w402) -> ("break ?"=w403:bool)
              }
            }
          }
          n232 = local read "Error Comment"() -> (w300:string)
          n233 = Not(x=w323) -> (.not. x?=w321:bool)
          n234 = Or(x=w321, y=w302) -> (x .or. y?=w322:bool)
          n235 = case shown="False" w322 {
            tunnel: w321 -> [_ w347]
            tunnel: w302 -> [w326 w343]
            tunnel: w319 -> [w332 w341]
            tunnel: w314 -> [w331 w340]
            tunnel: [w332 w338] -> w307
            tunnel: [w331 w339] -> w306
            tunnel: w303 -> [_ w337]
            tunnel: [w330 w335] -> w301
            tunnel: w300 -> [w330 w334]
            frame False {
              n236 = local read "Guiding"() -> (w329:bool)
              n237 = local read "Undo startguide"() -> (w328:bool)
              n238 = Compound Arithmetic op=AND(invert w326, w329, invert w328) -> (w327:bool)
              n239 = case shown="True" w327 {
                selector: w327 -> [_ w333]
                frame False {
                }
                frame True {
                  n240 = global write "Globals.vi" "StartGuide"(w333) -> ()
                }
              }
            }
            frame True {
              n241 = local read "Error code"() -> (w346:u8)
              n242 = case shown="False" w347 {
                tunnel: [w359 w370] -> w345
                tunnel: w346 -> [w359 w374]
                tunnel: w341 -> [w358 w369]
                tunnel: w340 -> [w357 w368]
                tunnel: [w357 w365] -> w339
                tunnel: [w358 w366] -> w338
                tunnel: w337 -> [_ w363]
                tunnel: [w356 w361] -> w336
                tunnel: w334 -> [w356 w360]
                frame False {
                }
                frame True {
                  n243 = call "EXCOM-CMD.vi"("VRN IN"=w369, "Bool Refnum"=w363, "Commande #"=13 ("NombredArguments"), "Error IN"=w368) -> ("VRN OUT"=w367:refnum<visa-resource-name>, "OK Done"=w372:bool, "Error OUT"=w364:errorcluster)  [unwired: 9 in]
                  n244 = Or(x=w374, y=u8 4) -> (x .or. y?=w371:u8)
                  n245 = case shown="False" w372 {
                    tunnel: w371 -> [w379 w386]
                    tunnel: [w378 w386] -> w370
                    tunnel: [w377 w385] -> w366
                    tunnel: w367 -> [w377 w385]
                    tunnel: [w376 w384] -> w365
                    tunnel: w364 -> [w376 w384]
                    frame False {
                      # "Ajoute le bit d'urgence !!!"
                      n246 = local read "Warning code"() -> (w381:u8)
                      n247 = Or(x=w381, y=u8 128) -> (x .or. y?=w382:u8)
                      n248 = Or(x=w379, y=u8 64) -> (x .or. y?=w378:u8)
                      n249 = local write "Warning code"(w382) -> ()
                    }
                    frame True {
                    }
                  }
                  n250 = Concatenate Strings(w360, "Attention, le télescope ne s'est pas arrêter !!!\n") -> (w361:string)
                }
              }
              n251 = case shown="False" w343 {
                tunnel: [w349 w354] -> w344
                tunnel: w345 -> [w349 w353]
                tunnel: w336 -> [w348 w351]
                tunnel: [w348 w350] -> w335
                frame False {
                }
                frame True {
                  n252 = Or(x=w353, y=u8 8) -> (x .or. y?=w354:u8)
                  n253 = Concatenate Strings(w351, "Attention, les tables n'ont pas atteintes leur position !!!\n") -> (w350:string)
                }
              }
              n254 = local write "Undo offset"(TRUE ("Undo offset")) -> ()
              n255 = local write "Error code"(w344) -> ()
            }
          }
          n256 = local read "VRN IN"() -> (w311:refnum<visa-resource-name>[])
          n257 = Replace Array Subset(array=w311, new element=w307, index=0) -> (w312:refnum<visa-resource-name>[])
          n258 = local write "Error Comment"(w301) -> ()
          n259 = local read "Error IN"() -> (w310:errorcluster[])
          n260 = local write "VRN IN"(w312) -> ()
          n261 = Replace Array Subset(array=w310, new element=w306, index=0) -> (w313:errorcluster[])
          n262 = local write "Error IN"(w313) -> ()
        }
        frame True {
        }
      }
    }
    frame #8 {
      # "Éventuellement, mettre un nombre d'itération de caméra au lieu d'un délai ...\nquoique, il faudrait voir comment tout ça s'harmonise avec un délai PCE ?!?"
      n263 = local read "Undo offset"() -> (w435:bool)
      n264 = local read "Guiding"() -> (w433:bool)
      n265 = Not(x=w435) -> (.not. x?=w434:bool)
      n266 = And(x=w434, y=w433) -> (x .and. y?=w432:bool)
      n267 = case shown="True" w432 {
        tunnel: w431 -> [_ w448]
        tunnel: w430 -> [_ w447]
        tunnel: [TRUE w446] -> w429
        frame False {
          # "Pas d'erreur de recentrage ..."
        }
        frame True {
          n268 = flat-sequence {
            tunnel: w447 -> [w450]
            tunnel: w448 -> [w449]
            tunnel: [w462] -> w446
            frame #0 {
              n269 = while {
                tunnel: w450 -> [w454]
                tunnel: w449 -> [w456]
                tunnel: [w451] -> _
                i -> [w460]
                stop <- w458 stop-if-true
                # "Attends 30 secondes que le guidage reparte ..."
                n270 = Wait (ms)(milliseconds to wait=u32 100) -> ()  [unwired: 1 out]
                n271 = Not Equal?(x=w454) -> (y=w455:sgl, x != y?=w453:bool)
                n272 = Not Equal?(y=w456) -> (x=w457:sgl, x != y?=w452:bool)
                n273 = Or(x=w453, y=w452) -> (x .or. y?=w451:bool)
                n274 = call "Max-iteration.vi"("i max"=300, "i act"=w460, "Valeur entrante"=w451) -> ("break ?"=w458:bool)
              }
            }
            frame #1 {
              n275 = while {
                tunnel: [w463] -> w462
                i -> [w466]
                stop <- w465 stop-if-true
                # "tolérance à réajuster"
                n276 = Wait Until Next ms Multiple(millisecond multiple=u32 100 ("n millisecondes")) -> ()  [unwired: 1 out]
                n277 = call-poly "Pytagore.vi"() -> ("Dist"=w474:dbl[], "Y"=w467:dbl[], "X"=w468:dbl[])
                n278 = Not Equal To 0?(x=w467) -> (x != 0?=w471:bool)
                n279 = Not Equal To 0?(x=w468) -> (x != 0?=w470:bool)
                n280 = Less?(x=w474, y=3.0) -> (x < y?=w469:bool[])
                n281 = Compound Arithmetic op=AND(w469, w470, w471) -> (w463:bool[])
                n282 = call "Max-iteration.vi"("i max"=300, "i act"=w466, "Valeur entrante"=w463) -> ("break ?"=w465:bool)
              }
            }
          }
        }
      }
      n283 = case shown="False" w429 {
        frame False {
          n284 = local read "Error Comment"() -> (w438:string)
          n285 = local read "Warning code"() -> (w442:u8)
          n286 = local read "Error code"() -> (w441:u8)
          n287 = Or(x=w441, y=u8 16) -> (x .or. y?=w440:u8)
          n288 = Or(x=w442, y=u8 16) -> (x .or. y?=w443:u8)
          n289 = Concatenate Strings(w438, "L'étoile ne s'est pas recentrée, peut-être pouvez-vous simplement attendre ?\n") -> (w437:string)
          n290 = local write "Warning code"(w443) -> ()
          n291 = local write "Error code"(w440) -> ()
          n292 = local write "Error Comment"(w437) -> ()
        }
        frame True {
        }
      }
    }
    frame #9 {
      # "Fermeture"
      n293 = local read "VRN IN"() -> (→"VRN OUT":refnum<visa-resource-name>[])
      n294 = local read "Error IN"() -> (→"Error OUT":errorcluster[])
    }
  }
